vi "XYZ-Measurement.vi"() -> ()   [LabVIEW 2011]
uses:
  <vilib>/Utility/file.llb/Write To Spreadsheet File (DBL).vi
  <vilib>/Analysis/NI_AALBase.lvlib
panel:
  in  "String":string
  out "Degauss in Process":bool
  in  "phi":dbl
  in  "theta (xy-ebene)":dbl
  in  "VISA-Ressourcenname":refnum<visa-resource-name>="COM7"
  out "Data":T1
  in  "z":dbl=0.065
  in  "x":dbl=0.115
  in  "y":dbl=-0.158
  in  "Magnitude_Step_Size":dbl
  in  "Magnitude_End":dbl
  in  "Magnitude_Start":dbl
  out "DeviceID":u8 format="%02x"
  out "Z_Range":dbl
  out "X_Y_Range":dbl
  in  "iIndex":u32
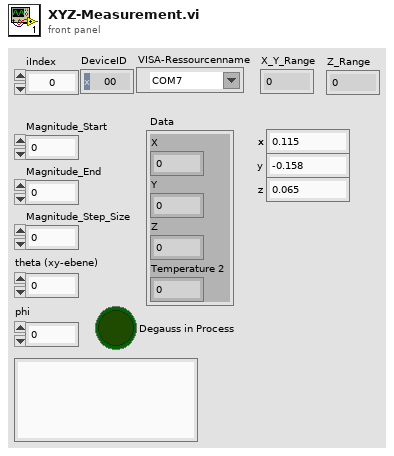
[diagram p1: front panel]
types:
  T1 = cluster{"X":dbl, "Y":dbl, "Z":dbl, "Temperature 2":dbl}
  T2 = enum8{"Standard I2C 3-byte read command", "1-byte I2C read command for 16bit sensor data and conversion\nstatus", "1-byte I2C read command for 8 bit sensor MSB data and\nconversion status", "Reserved"}
  T3 = enum8{"Enabled", "Disabled", "Disabled and Grayed Out"}
  T4 = cluster{"Temperature (°C)":dbl, "x (mT)":dbl, "y (mT)":dbl, "z (mT)":dbl}
  T5 = cluster{"I2C_RD":enum8{"Standard I2C 3-byte read command", "1-byte I2C read command for 16bit sensor data and conversion\nstatus", "1-byte I2C read command for 8 bit sensor MSB data and\nconversion status", "Reserved"}, "CONV_AVG":enum8{"1x average, 10.0-kSPS (3-axes) or 20-kSPS (1 axis)", "2x average, 5.7-kSPS (3-axes) or 13.3-kSPS (1 axis)", "4x average, 3.1-kSPS (3-axes) or 8.0-kSPS (1 axis)", "8x average, 1.6-kSPS (3-axes) or 4.4-kSPS (1 axis)", "16x average, 0.8-kSPS (3-axes) or 2.4-kSPS (1 axis)", "32x average, 0.4-kSPS (3-axes) or 1.2-kSPS (1 axis)"}, "MAG_TEMPCO":enum8{"0 %/°C (No temperature compensation)", "0.12 %/°C (NdBFe)", "0.03 %/°C (SmCo)", "0.20 %/°C (Ceramic)"}, "CRC_EN":enum8{"CRC disabled", "CRC enabled"}}
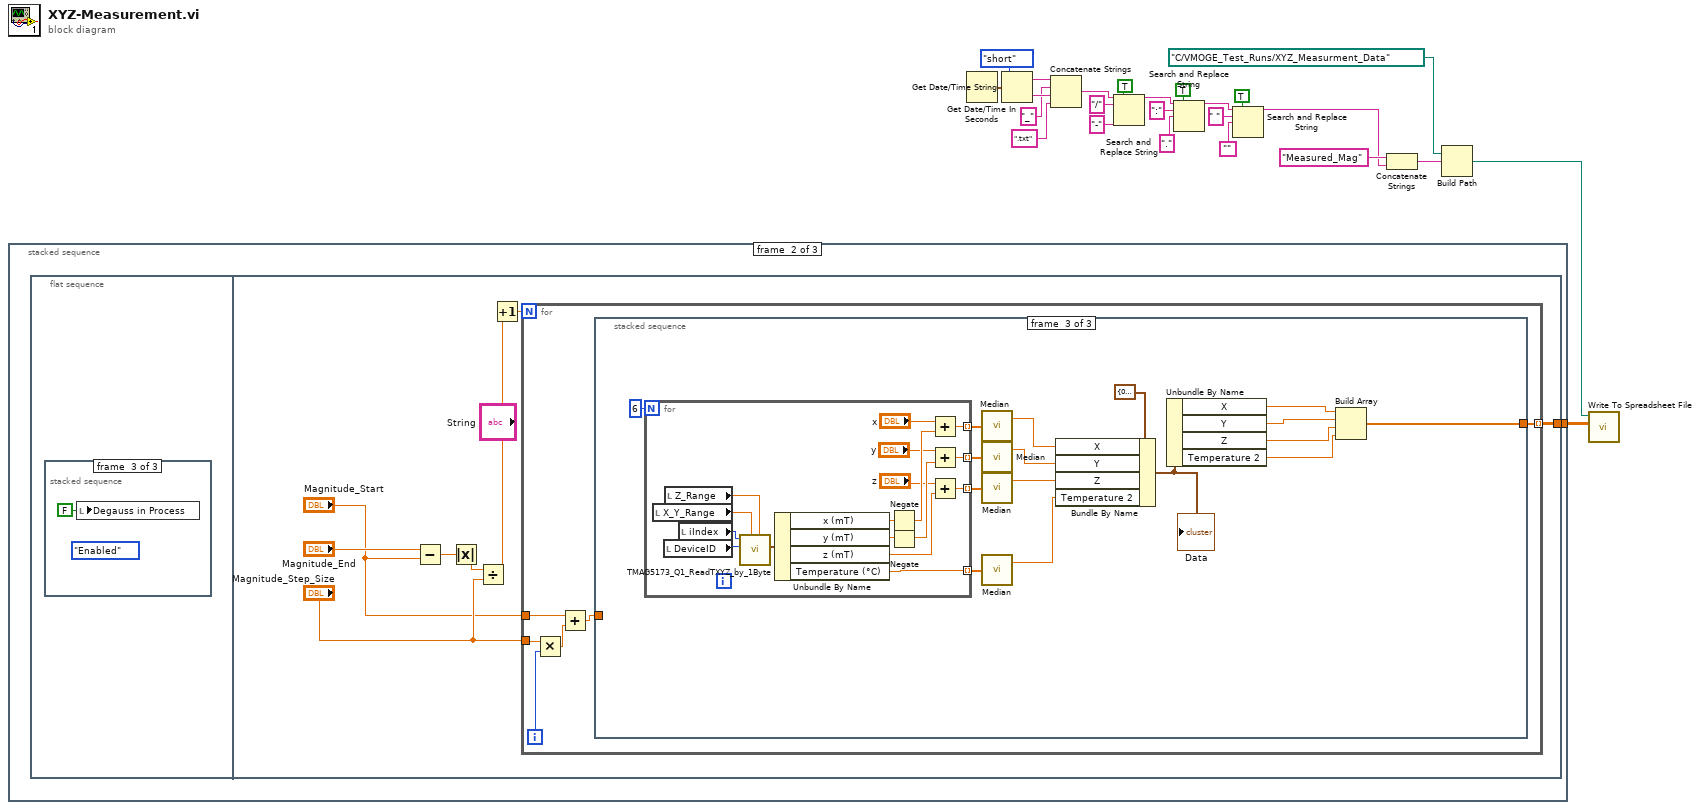
[diagram p0: block diagram]
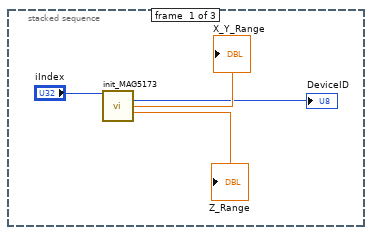
[diagram p2: hidden frame]
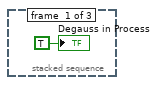
[diagram p3: hidden frame]
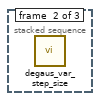
[diagram p4: hidden frame]
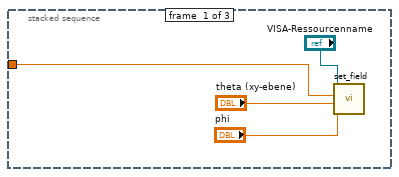
[diagram p5: hidden frame]
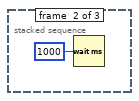
[diagram p6: hidden frame]
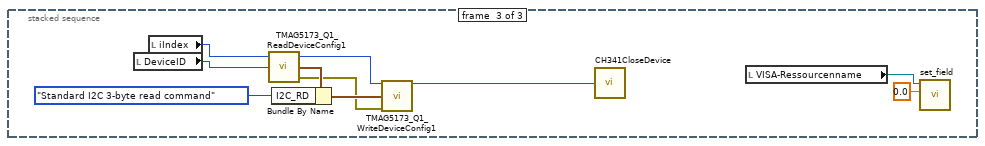
[diagram p7: hidden frame]
diagram:
  n1 = stacked-sequence {
    tunnel: [_ w29 _] -> w2
    frame #0 {
      n2 = call "init_MAG5173.vi"("iIndex"="iIndex") -> ("DeviceID"=→"DeviceID":u8, "X_Y_Range"=→"X_Y_Range":dbl, "Z_Range"=→"Z_Range":dbl)  [unwired: 10 in, 2 out]
    }
    frame #1 {
      n3 = flat-sequence {
        tunnel: [w32] -> w29
        frame #0 {
          n4 = stacked-sequence {
            frame #0 {
              "Degauss in Process" <- TRUE ("Degauss in Process")
            }
            frame #1 {
              n5 = call "degaus_var_step_size.vi"() -> ()  [unwired: 12 in]
            }
            frame #2 {
              (unwired) T3."Enabled" ("Disabled")
              n6 = local write "Degauss in Process"(FALSE ("Degauss in Process")) -> ()
            }
          }
        }
        frame #1 {
          n7 = Subtract(x="Magnitude_End", y="Magnitude_Start") -> (x-y=w39:dbl)
          n8 = Absolute Value(x=w39) -> (abs(x)=w38:dbl)
          n9 = Divide(x=w38, y="Magnitude_Step_Size") -> (x/y=w37:dbl)
          n10 = Increment(x=w37) -> (x+1=w35:dbl)
          n11 = for {
            N: w35 -> [_]
            tunnel: "Magnitude_Step_Size" -> [w44]
            tunnel: "Magnitude_Start" -> [w43]
            tunnel: [w40] -> w32 mode=indexing
            i -> [w45]
            n12 = Multiply(x=w44, y=w45) -> (x*y=w42:dbl)
            n13 = Add(x=w43, y=w42) -> (x+y=w41:dbl)
            n14 = stacked-sequence {
              tunnel: w41 -> [w46 _ _]
              tunnel: [_ _ w52] -> w40
              frame #0 {
                n15 = call "set_field.vi"("phi"="phi", "theta (xy-ebene)"="theta (xy-ebene)", "Magnitude (mT)"=w46, "VISA-Ressourcenname"="VISA-Ressourcenname") -> ()  [unwired: 8 in]
              }
              frame #1 {
                n16 = Wait (ms)(milliseconds to wait=u32 1000) -> ()  [unwired: 1 out]
              }
              frame #2 {
                n17 = for {
                  N: 6 -> [_]
                  tunnel: [w75] -> w64 mode=indexing
                  tunnel: [w74] -> w65 mode=indexing
                  tunnel: [w73] -> w66 mode=indexing
                  tunnel: [w72] -> w63 mode=indexing
                  n18 = local read "X_Y_Range"() -> (w68:dbl)
                  n19 = local read "DeviceID"() -> (w82:u8)
                  n20 = local read "Z_Range"() -> (w67:dbl)
                  n21 = local read "iIndex"() -> (w83:u32)
                  n22 = call <userlib>:"TMAG5173_Q1_ReadTXYZ_by_1Byte.vi"("z-Range"=w67, "xy-Range"=w68, "DeviceID"=w82, "iIndex"=w83) -> ("Data"=w81:T4)  [unwired: 4 in, 3 out]
                  n23 = Unbundle By Name(w81) -> ("x (mT)"=w80:dbl, "y (mT)"=w79:dbl, "z (mT)"=w76:dbl, "Temperature (°C)"=w72:dbl)
                  n24 = Negate(x=w80) -> (-x=w77:dbl)
                  n25 = Negate(x=w79) -> (-x=w78:dbl)
                  n26 = Add(x="x", y=w77) -> (x+y=w75:dbl)
                  n27 = Add(x="y", y=w78) -> (x+y=w74:dbl)
                  n28 = Add(x="z", y=w76) -> (x+y=w73:dbl)
                }
                n29 = call <vilib>:"Median.vi"("X"=w64) -> ("median"=w62:dbl)  [unwired: 1 out]
                n30 = call <vilib>:"Median.vi"("X"=w65) -> ("median"=w61:dbl)  [unwired: 1 out]
                n31 = call <vilib>:"Median.vi"("X"=w66) -> ("median"=w60:dbl)  [unwired: 1 out]
                n32 = call <vilib>:"Median.vi"("X"=w63) -> ("median"=w57:dbl)  [unwired: 1 out]
                n33 = Bundle By Name(cluster=T1 {"X"=0.0, "Y"=0.0, "Z"=0.0, "Temperature 2"=0.0} ("data"), "X"=w62, "Y"=w61, "Z"=w60, "Temperature 2"=w57) -> (w56:T1)
                "Data" <- w56
                n34 = Unbundle By Name(w56) -> ("X"=w55:dbl, "Y"=w54:dbl, "Z"=w53:dbl, "Temperature 2"=w51:dbl)
                n35 = Build Array(w55, w54, w53, w51) -> (w52:dbl[])
              }
            }
          }
        }
      }
    }
    frame #2 {
      n36 = local read "DeviceID"() -> (w87:u8)
      n37 = local read "iIndex"() -> (w88:u32)
      n38 = call <userlib>:"TMAG5173_Q1_ReadDeviceConfig1.vi"("DeviceID"=w87, "iIndex"=w88) -> ("error out"=w89:errorcluster, "Device_Config_1"=w93:T5, "oIndex"=w90:u32)  [unwired: 1 in]
      n39 = Bundle By Name(cluster=w93, "I2C_RD"=T2."Standard I2C 3-byte read command") -> (w92:T5)
      n40 = call <userlib>:"TMAG5173_Q1_WriteDeviceConfig1.vi"("iIndex"=w90, "Device_Config_1"=w92, "error in (no error)"=w89) -> ("oIndex"=w86:u32)  [unwired: 10 in, 2 out]
      n41 = call <userlib>:"CH341CloseDevice.vi"("iIndex"=w86) -> ()  [unwired: 1 in]
      n42 = local read "VISA-Ressourcenname"() -> (w84:refnum<visa-resource-name>)
      n43 = call "set_field.vi"("Magnitude (mT)"=0.0, "VISA-Ressourcenname"=w84) -> ()  [unwired: 10 in]
    }
  }
  n44 = Get Date/Time In Seconds() -> (seconds since 1Jan1904=w22:timestamp)
  n45 = Get Date/Time String(date format (0)=enum16{"short", "long", "abbreviated"}."short", seconds (now)=w22) -> (date string=w20:string, time string=w16:string)  [unwired: 1 in]
  n46 = Concatenate Strings(w20, "_" ("string"), w16, ".txt" ("string")) -> (w19:string)
  n47 = Search and Replace String(replace all?=TRUE ("replace all? (F)"), input string=w19, search string="/", replace string="-" ("replace string (\"\")")) -> (result string=w13:string)  [unwired: 4 in, 3 out]
  n48 = Search and Replace String(replace all?=TRUE ("replace all? (F)"), input string=w13, search string=":", replace string="." ("replace string (\"\")")) -> (result string=w9:string)  [unwired: 4 in, 3 out]
  n49 = Search and Replace String(replace all?=TRUE ("replace all? (F)"), input string=w9, search string=" ", replace string="") -> (result string=w4:string)  [unwired: 4 in, 3 out]
  n50 = Concatenate Strings("Measured_Mag" ("name or relative path"), w4) -> (w23:string)
  n51 = Build Path(base path=path "C:/VMOGE_Test_Runs/XYZ_Measurment_Data" ("file path (dialog if empty)"), name or relative path=w23) -> (appended path=w1:path)
  n52 = call-poly <vilib>:"Write To Spreadsheet File.vi"("2D data"=w2, "file path (dialog if empty)"=w1) -> ()  [unwired: 6 in, 1 out]
